vi "test_read-nmea-data2.vi"() -> ()   [LabVIEW 2019] (continued)
F9P\t$GBGSV,1,1,03,11,50,132,,14,87,127,,33,60,219,,3*40\n\t\n15:11:56.71\tF9P\t$GNGLL,3723.52845,N,12656.92271,E,061158.00,A,A*7E\n\t\n15:11:56.73\tF9P\t\t\n15:11:56.75\tF9P\t\t\n15:11:56.77\tF9P\t\t\n15:11:56.79\tF9P\t\t\n15:11:56.81\tF9P\t\t\n15:11:56.83\tF9P\t\t\n15:11:56.85\tF9P\t\t\n15:11:56.87\tF9P\t\t\n15:11:56.89\tF9P\t\t\n15:11:56.91\tF9P\t\t\n15:11:56.93\tF9P\t\t\n15:11:56.95\tF9P\t\t\n15:11:56.97\tF9P\t\t\n15:11:56.99\tF9P\t\t\n15:11:57.01\tF9P\t\t\n15:11:57.03\tF9P\t\t\n15:11:57.05\tF9P\t\t\n15:11:57.07\tF9P\t\t\n15:11:57.09\tF9P\t\t\n15:11:57.11\tF9P\t\t\n15:11:57.13\tF9P\t\t\n15:11:57.15\tF9P\t\t\n15:11:57.17\tF9P\t\t\n15:11:57.19\tF9P\t\t\n15:11:57.21\tF9P\t\t\n15:11:57.23\tF9P\t\t\n15:11:57.25\tF9P\t$GNRMC,061159.00,A,3723.52891,N,12656.92353,E,2.815,44.65,250720,,,A,V*35\n\t\n15:11:57.27\tF9P\t$GNVTG,44.65,T,,M,2.815,N,5.213,K,A*1B\n\t\n15:11:57.29\tF9P\t$GNGGA,061159.00,3723.52891,N,12656.92353,E,1,12,0.67,33.2,M,18.5,M,,*7E\n\t\n15:11:57.31\tF9P\t$GNGSA,A,3,12,06,19,05,17,09,04,02,,,,,1.25,0.67,1.05,1*03\n\t\n15:11:57.33\tF9P\t$GNGSA,A,3,85,70,71,84,,,,,,,,,1.25,0.67,1.05,2*01\n\t\n15:11:57.35\tF9P\t$GNGSA,A,3,36,19,11,04,09,12,,,,,,,1.25,0.67,1.05,3*03\n\t\n15:11:57.37\tF9P\t$GNGSA,A,3,14,11,33,,,,,,,,,,1.25,0.67,1.05,4*02\n\t\n15:11:57.39\tF9P\t$GPGSV,3,1,09,02,55,319,44,04,18,043,20,05,37,247,31,06,64,049,32,1*64\n\t\n15:11:57.41\tF9P\t$GPGSV,3,2,09,09,45,074,39,12,24,277,26,17,33,153,36,19,53,157,32,1*66\n\t\n15:11:57.43\tF9P\t$GPGSV,3,3,09,25,12,307,15,1*59\n\t\n15:11:57.45\tF9P\t$GPGSV,3,1,09,02,55,319,,04,18,043,15,05,37,247,15,06,64,049,26,6*66\n\t\n15:11:57.47\tF9P\t$GPGSV,3,2,09,09,45,074,27,12,24,277,12,17,33,153,25,19,53,157,,6*6A\n\t\n15:11:57.49\tF9P\t$GPGSV,3,3,09,25,12,307,,6*5A\n\t\n15:11:57.51\tF9P\t$GLGSV,2,1,08,69,12,031,,70,71,039,32,71,52,205,43,72,04,209,,1*7C\n\t\n15:11:57.53\tF9P\t$GLGSV,2,2,08,77,01,326,,84,20,122,11,85,70,067,39,86,37,330,,1*72\n\t\n15:11:57.55\tF9P\t$GLGSV,2,1,08,69,12,031,,70,71,039,,71,52,205,28,72,04,209,,3*72\n\t\n15:11:57.57\tF9P\t$GLGSV,2,2,08,77,01,326,,84,20,122,18,85,70,067,24,86,37,330,,3*75\n\t\n15:11:57.59\tF9P\t$GAGSV,2,1,08,02,08,297,10,04,66,118,33,09,32,193,30,11,71,358,24,7*7D\n\t\n15:11:57.61\tF9P\t$GAGSV,2,2,08,12,40,102,31,19,26,045,31,25,09,249,,36,26,308,28,7*73\n\t\n15:11:57.63\tF9P\t$GAGSV,2,1,08,02,08,297,,04,66,118,,09,32,193,26,11,71,358,,2*78\n\t\n15:11:57.65\tF9P\t$GAGSV,2,2,08,12,40,102,,19,26,045,,25,09,249,,36,26,308,,2*7C\n\t\n15:11:57.67\tF9P\t$GBGSV,1,1,03,11,50,132,29,14,87,127,31,33,60,219,38,1*40\n\t\n15:11:57.69\tF9P\t$GBGSV,1,1,03,11,50,132,,14,87,127,31,33,60,219,,3*42\n\t\n15:11:57.71\tF9P\t$GNGLL,3723.52891,N,12656.92353,E,061159.00,A,A*77\n\t\n15:11:57.73\tF9P\t\t\n15:11:57.75\tF9P\t\t\n15:11:57.77\tF9P\t\t\n15:11:57.79\tF9P\t\t\n15:11:57.81\tF9P\t\t\n15:11:57.83\tF9P\t\t\n15:11:57.85\tF9P\t\t\n15:11:57.87\tF9P\t\t\n15:11:57.89\tF9P\t\t\n15:11:57.91\tF9P\t\t\n15:11:57.93\tF9P\t\t\n15:11:57.95\tF9P\t\t\n15:11:57.97\tF9P\t\t\n15:11:57.99\tF9P\t\t\n15:11:58.01\tF9P\t\t\n15:11:58.03\tF9P\t\t\n15:11:58.05\tF9P\t\t\n15:11:58.07\tF9P\t\t\n15:11:58.09\tF9P\t\t\n15:11:58.11\tF9P\t\t\n15:11:58.13\tF9P\t\t\n15:11:58.15\tF9P\t\t\n15:11:58.17\tF9P\t\t\n15:11:58.19\tF9P\t\t\n15:11:58.21\tF9P\t\t\n15:11:58.23\tF9P\t\t\n15:11:58.25\tF9P\t$GNRMC,061200.00,A,3723.52933,N,12656.92401,E,2.063,43.37,250720,,,A,V*3A\n\t\n15:11:58.27\tF9P\t$GNVTG,43.37,T,,M,2.063,N,3.820,K,A*1E\n\t\n15:11:58.29\tF9P\t$GNGGA,061200.00,3723.52933,N,12656.92401,E,1,12,0.68,33.6,M,18.5,M,,*73\n\t\n15:11:58.31\tF9P\t$GNGSA,A,3,12,06,19,05,17,09,04,02,,,,,1.27,0.68,1.07,1*0C\n\t\n15:11:58.33\tF9P\t$GNGSA,A,3,85,70,71,84,,,,,,,,,1.27,0.68,1.07,2*0E\n\t\n15:11:58.35\tF9P\t$GNGSA,A,3,36,19,11,04,09,12,,,,,,,1.27,0.68,1.07,3*0C\n\t\n15:11:58.37\tF9P\t$GNGSA,A,3,14,11,33,,,,,,,,,,1.27,0.68,1.07,4*0D\n\t\n15:11:58.39\tF9P\t$GPGSV,3,1,09,02,55,319,43,04,18,043,20,05,37,247,28,06,64,049,30,1*69\n\t\n15:11:58.41\tF9P\t$GPGSV,3,2,09,09,45,074,37,12,24,277,25,17,33,153,28,19,53,157,31,1*67\n\t\n15:11:58.43\tF9P\t$GPGSV,3,3,09,25,12,307,17,1*5B\n\t\n15:11:58.45\tF9P\t$GPGSV,3,1,09,02,55,319,,04,18,043,14,05,37,247,14,06,64,049,26,6*66\n\t\n15:11:58.47\tF9P\t$GPGSV,3,2,09,09,45,074,27,12,24,277,14,17,33,153,25,19,53,157,,6*6C\n\t\n15:11:58.49\tF9P\t$GPGSV,3,3,09,25,12,307,,6*5A\n\t\n15:11:58.51\tF9P\t$GLGSV,2,1,08,69,12,031,,70,71,039,31,71,52,205,40,72,04,209,,1*7C\n\t\n15:11:58.53\tF9P\t$GLGSV,2,2,08,77,01,326,,84,20,122,10,85,70,067,36,86,37,330,,1*7C\n\t\n15:11:58.55\tF9P\t$GLGSV,2,1,08,69,12,031,,70,71,039,,71,52,205,26,72,04,209,,3*7C\n\t\n15:11:58.57\tF9P\t$GLGSV,2,2,08,77,01,326,,84,20,122,16,85,70,067,23,86,37,330,,3*7C\n\t\n15:11:58.59\tF9P\t$GAGSV,2,1,08,02,08,297,10,04,66,118,33,09,32,193,31,11,71,358,31,7*78\n\t\n15:11:58.61\tF9P\t$GAGSV,2,2,08,12,40,102,31,19,26,045,30,25,09,249,,36,26,308,27,7*7D\n\t\n15:11:58.63\tF9P\t$GAGSV,2,1,08,02,08,297,,04,66,118,,09,32,193,,11,71,358,,2*7C\n\t\n15:11:58.65\tF9P\t$GAGSV,2,2,08,12,40,102,,19,26,045,,25,09,249,,36,26,308,,2*7C\n\t\n15:11:58.67\tF9P\t$GBGSV,1,1,03,11,50,132,28,14,87,127,28,33,60,219,40,1*46\n\t\n15:11:58.69\tF9P\t$GBGSV,1,1,03,11,50,132,,14,87,127,30,33,60,219,,3*43\n\t\n15:11:58.71\tF9P\t$GNGLL,3723.52933,N,12656.92401,E,061200.00,A,A*71\n\t\n15:11:58.73\tF9P\t\t\n15:11:58.75\tF9P\t\t\n15:11:58.77\tF9P\t\t\n15:11:58.79\tF9P\t\t\n15:11:58.81\tF9P\t\t\n15:11:58.83\tF9P\t\t\n15:11:58.85\tF9P\t\t\n15:11:58.87\tF9P\t\t\n15:11:58.89\tF9P\t\t\n15:11:58.91\tF9P\t\t\n15:11:58.93\tF9P\t\t\n15:11:58.95\tF9P\t\t\n15:11:58.97\tF9P\t\t\n15:11:58.99\tF9P\t\t\n15:11:59.01\tF9P\t\t\n15:11:59.03\tF9P\t\t\n15:11:59.05\tF9P\t\t\n15:11:59.07\tF9P\t\t\n15:11:59.09\tF9P\t\t\n15:11:59.11\tF9P\t\t\n15:11:59.13\tF9P\t\t\n15:11:59.15\tF9P\t\t\n15:11:59.17\tF9P\t\t\n15:11:59.19\tF9P\t\t\n15:11:59.21\tF9P\t\t\n15:11:59.23\tF9P\t\t\n15:11:59.25\tF9P\t$GNRMC,061201.00,A,3723.52964,N,12656.92469,E,2.580,59.46,250720,,,A,V*32\n\t\n15:11:59.27\tF9P\t$GNVTG,59.46,T,,M,2.580,N,4.779,K,A*1F\n\t\n15:11:59.29\tF9P\t$GNGGA,061201.00,3723.52964,N,12656.92469,E,1,12,0.73,33.3,M,18.5,M,,*71\n\t\n15:11:59.32\tF9P\t$GNGSA,A,3,12,06,19,05,17,09,02,,,,,,1.41,0.73,1.20,1*07\n\t\n15:11:59.34\tF9P\t$GNGSA,A,3,85,70,71,84,,,,,,,,,1.41,0.73,1.20,2*01\n\t\n15:11:59.36\tF9P\t$GNGSA,A,3,36,19,11,04,09,12,,,,,,,1.41,0.73,1.20,3*03\n\t\n15:11:59.38\tF9P\t$GNGSA,A,3,14,11,33,,,,,,,,,,1.41,0.73,1.20,4*02\n\t\n15:11:59.40\tF9P\t$GPGSV,3,1,09,02,55,319,41,04,18,043,19,05,37,247,27,06,64,049,25,1*6A\n\t\n15:11:59.42\tF9P\t$GPGSV,3,2,09,09,45,074,32,12,24,277,24,17,33,153,36,19,53,157,27,1*6B\n\t\n15:11:59.44\tF9P\t$GPGSV,3,3,09,25,12,307,15,1*59\n\t\n15:11:59.46\tF9P\t$GPGSV,3,1,09,02,55,319,,04,18,043,,05,37,247,,06,64,049,24,6*64\n\t\n15:11:59.48\tF9P\t$GPGSV,3,2,09,09,45,074,27,12,24,277,14,17,33,153,23,19,53,157,,6*6A\n\t\n15:11:59.50\tF9P\t$GPGSV,3,3,09,25,12,307,,6*5A\n\t\n15:11:59.52\tF9P\t$GLGSV,2,1,08,69,12,031,,70,71,039,25,71,52,205,44,72,04,209,,1*7D\n\t\n15:11:59.54\tF9P\t$GLGSV,2,2,08,77,01,326,,84,20,122,14,85,70,067,29,86,37,330,,1*76\n\t\n15:11:59.56\tF9P\t$GLGSV,2,1,08,69,12,031,,70,71,039,,71,52,205,26,72,04,209,,3*7C\n\t\n15:11:59.58\tF9P\t$GLGSV,2,2,08,77,01,326,,84,20,122,11,85,70,067,21,86,37,330,,3*79\n\t\n15:11:59.60\tF9P\t$GAGSV,2,1,08,02,08,297,09,04,66,118,30,09,32,193,35,11,71,358,34,7*72\n\t\n15:11:59.62\tF9P\t$GAGSV,2,2,08,12,40,102,31,19,26,045,29,25,09,249,,36,26,308,26,7*74\n\t\n15:11:59.64\tF9P\t$GAGSV,2,1,08,02,08,297,,04,66,118,,09,32,193,,11,71,358,,2*7C\n\t\n15:11:59.66\tF9P\t$GAGSV,2,2,08,12,40,102,,19,26,045,,25,09,249,,36,26,308,,2*7C\n\t\n15:11:59.68\tF9P\t$GBGSV,1,1,03,11,50,132,20,14,87,127,28,33,60,219,39,1*40\n\t\n15:11:59.70\tF9P\t$GBGSV,1,1,03,11,50,132,,14,87,127,31,33,60,219,,3*42\n\t\n15:11:59.72\tF9P\t$GNGLL,3723.52964,N,12656.92469,E,061201.00,A,A*7C\n\t\n15:11:59.74\tF9P\t\t\n15:11:59.76\tF9P\t\t\n15:11:59.78\tF9P\t\t\n15:11:59.80\tF9P\t\t\n15:11:59.82\tF9P\t\t\n15:11:59.84\tF9P\t\t\n15:11:59.86\tF9P\t\t\n15:11:59.88\tF9P\t\t\n15:11:59.90\tF9P\t\t\n15:11:59.92\tF9P\t\t\n15:11:59.94\tF9P\t\t\n15:11:59.96\tF9P\t\t\n15:11:59.98\tF9P\t\t\n15:12:00.00\tF9P\t\t\n15:12:00.02\tF9P\t\t\n15:12:00.04\tF9P\t\t\n15:12:00.06\tF9P\t\t\n15:12:00.08\tF9P\t\t\n15:12:00.10\tF9P\t\t\n15:12:00.12\tF9P\t\t\n15:12:00.14\tF9P\t\t\n15:12:00.16\tF9P\t\t\n15:12:00.18\tF9P\t\t\n15:12:00.20\tF9P\t\t\n15:12:00.22\tF9P\t\t\n15:12:00.24\tF9P\t\t\n15:12:00.26\tF9P\t$GNRMC,061202.00,A,3723.53000,N,12656.92524,E,2.015,53.71,250720,,,A,V*34\n\t\n15:12:00.28\tF9P\t$GNVTG,53.71,T,,M,2.015,N,3.732,K,A*10\n\t\n15:12:00.30\tF9P\t$GNGGA,061202.00,3723.53000,N,12656.92524,E,1,12,0.70,33.1,M,18.5,M,,*71\n\t\n15:12:00.32\tF9P\t$GNGSA,A,3,12,06,19,05,17,09,04,02,,,,,1.27,0.70,1.06,1*04\n\t\n15:12:00.34\tF9P\t$GNGSA,A,3,85,70,71,84,,,,,,,,,1.27,0.70,1.06,2*06\n\t\n15:12:00.36\tF9P\t$GNGSA,A,3,36,19,11,04,09,12,,,,,,,1.27,0.70,1.06,3*04\n\t\n15:12:00.38\tF9P\t$GNGSA,A,3,14,11,33,,,,,,,,,,1.27,0.70,1.06,4*05\n\t\n15:12:00.40\tF9P\t$GPGSV,3,1,09,02,55,319,43,04,18,043,21,05,37,247,26,06,64,049,31,1*67\n\t\n15:12:00.42\tF9P\t$GPGSV,3,2,09,09,45,074,35,12,24,277,27,17,33,153,37,19,53,157,28,1*61\n\t\n15:12:00.44\tF9P\t$GPGSV,3,3,09,25,12,307,15,1*59\n\t\n15:12:00.46\tF9P\t$GPGSV,3,1,09,02,55,319,,04,18,043,,05,37,247,,06,64,049,23,6*63\n\t\n15:12:00.48\tF9P\t$GPGSV,3,2,09,09,45,074,27,12,24,277,11,17,33,153,23,19,53,157,,6*6F\n\t\n15:12:00.50\tF9P\t$GPGSV,3,3,09,25,12,307,,6*5A\n\t\n15:12:00.52\tF9P\t$GLGSV,2,1,08,69,12,031,,70,71,039,26,71,52,205,42,72,04,209,28,1*72\n\t\n15:12:00.54\tF9P\t$GLGSV,2,2,08,77,01,326,,84,20,122,08,85,70,067,34,86,37,330,,1*77\n\t\n15:12:00.56\tF9P\t$GLGSV,2,1,08,69,12,031,,70,71,039,,71,52,205,25,72,04,209,,3*7F\n\t\n15:12:00.58\tF9P\t$GLGSV,2,2,08,77,01,326,,84,20,122,11,85,70,067,21,86,37,330,,3*79\n\t\n15:12:00.60\tF9P\t$GAGSV,2,1,08,02,08,297,13,04,66,118,33,09,32,193,36,11,71,358,26,7*7A\n\t\n15:12:00.62\tF9P\t$GAGSV,2,2,08,12,40,102,27,19,26,045,28,25,09,249,,36,26,308,25,7*71\n\t\n15:12:00.64\tF9P\t$GAGSV,2,1,08,02,08,297,,04,66,118,,09,32,193,,11,71,358,,2*7C\n\t\n15:12:00.66\tF9P\t$GAGSV,2,2,08,12,40,102,,19,26,045,,25,09,249,,36,26,308,,2*7C\n\t\n15:12:00.68\tF9P\t$GBGSV,1,1,03,11,50,132,31,14,87,127,28,33,60,219,40,1*4E\n\t\n15:12:00.70\tF9P\t$GBGSV,1,1,03,11,50,132,,14,87,127,28,33,60,219,,3*4A\n\t\n15:12:00.72\tF9P\t$GNGLL,3723.53000,N,12656.92524,E,061202.00,A,A*7D\n\t\n15:12:00.74\tF9P\t\t\n15:12:00.76\tF9P\t\t\n15:12:00.78\tF9P\t\t\n15:12:00.80\tF9P\t\t\n15:12:00.82\tF9P\t\t\n15:12:00.84\tF9P\t\t\n15:12:00.86\tF9P\t\t\n15:12:00.88\tF9P\t\t\n15:12:00.90\tF9P\t\t\n15:12:00.92\tF9P\t\t\n15:12:00.94\tF9P\t\t\n15:12:00.96\tF9P\t\t\n15:12:00.98\tF9P\t\t\n15:12:01.00\tF9P\t\t\n15:12:01.02\tF9P\t\t\n15:12:01.04\tF9P\t\t\n15:12:01.06\tF9P\t\t\n15:12:01.08\tF9P\t\t\n15:12:01.10\tF9P\t\t\n15:12:01.12\tF9P\t\t\n15:12:01.14\tF9P\t\t\n15:12:01.16\tF9P\t\t\n15:12:01.18\tF9P\t\t\n15:12:01.20\tF9P\t\t\n15:12:01.22\tF9P\t\t\n15:12:01.24\tF9P\t\t\n15:12:01.26\tF9P\t$GNRMC,061203.00,A,3723.53041,N,12656.92573,E,2.202,48.58,250720,,,A,V*37\n\t\n15:12:01.28\tF9P\t$GNVTG,48.58,T,,M,2.202,N,4.077,K,A*14\n\t\n15:12:01.30\tF9P\t$GNGGA,061203.00,3723.53041,N,12656.92573,E,1,12,0.70,33.4,M,18.5,M,,*72\n\t\n15:12:01.32\tF9P\t$GNGSA,A,3,12,06,19,05,17,09,04,02,,,,,1.27,0.70,1.06,1*04\n\t\n15:12:01.34\tF9P\t$GNGSA,A,3,85,70,71,84,,,,,,,,,1.27,0.70,1.06,2*06\n\t\n15:12:01.36\tF9P\t$GNGSA,A,3,36,19,11,04,09,12,,,,,,,1.27,0.70,1.06,3*04\n\t\n15:12:01.38\tF9P\t$GNGSA,A,3,14,11,33,,,,,,,,,,1.27,0.70,1.06,4*05\n\t\n15:12:01.40\tF9P\t$GPGSV,3,1,09,02,55,319,42,04,18,043,21,05,37,247,30,06,64,049,30,1*60\n\t\n15:12:01.42\tF9P\t$GPGSV,3,2,09,09,45,074,33,12,24,277,27,17,33,153,32,19,53,157,30,1*6B\n\t\n15:12:01.44\tF9P\t$GPGSV,3,3,09,25,12,307,12,1*5E\n\t\n15:12:01.46\tF9P\t$GPGSV,3,1,09,02,55,319,,04,18,043,,05,37,247,,06,64,049,23,6*63\n\t\n15:12:01.48\tF9P\t$GPGSV,3,2,09,09,45,074,32,12,24,277,12,17,33,153,23,19,53,157,,6*68\n\t\n15:12:01.50\tF9P\t$GPGSV,3,3,09,25,12,307,,6*5A\n\t\n15:12:01.52\tF9P\t$GLGSV,2,1,08,69,12,031,,70,71,039,27,71,52,205,44,72,04,209,20,1*7D\n\t\n15:12:01.54\tF9P\t$GLGSV,2,2,08,77,01,326,,84,20,122,11,85,70,067,28,86,37,330,,1*72\n\t\n15:12:01.56\tF9P\t$GLGSV,2,1,08,69,12,031,,70,71,039,,71,52,205,26,72,04,209,,3*7C\n\t\n15:12:01.58\tF9P\t$GLGSV,2,2,08,77,01,326,,84,20,122,08,85,70,067,21,86,37,330,,3*71\n\t\n15:12:01.60\tF9P\t$GAGSV,2,1,08,02,08,297,11,04,66,118,29,09,32,193,37,11,71,358,31,7*74\n\t\n15:12:01.62\tF9P\t$GAGSV,2,2,08,12,40,102,26,19,26,045,28,25,09,249,,36,26,308,23,7*76\n\t\n15:12:01.64\tF9P\t$GAGSV,2,1,08,02,08,297,,04,66,118,,09,32,193,28,11,71,358,,2*76\n\t\n15:12:01.66\tF9P\t$GAGSV,2,2,08,12,40,102,,19,26,045,,25,09,249,,36,26,308,,2*7C\n\t\n15:12:01.68\tF9P\t$GBGSV,1,1,03,11,50,132,25,14,87,127,26,33,60,219,35,1*47\n\t\n15:12:01.70\tF9P\t$GBGSV,1,1,03,11,50,132,,14,87,127,27,33,60,219,,3*45\n\t\n15:12:01.72\tF9P\t$GNGLL,3723.53041,N,12656.92573,E,061203.00,A,A*7B\n\t\n15:12:01.74\tF9P\t\t\n15:12:01.76\tF9P\t\t\n15:12:01.78\tF9P\t\t\n15:12:01.80\tF9P\t\t\n15:12:01.82\tF9P\t\t\n15:12:01.84\tF9P\t\t\n15:12:01.86\tF9P\t\t\n15:12:01.88\tF9P\t\t\n15:12:01.90\tF9P\t\t\n15:12:01.92\tF9P\t\t\n15:12:01.94\tF9P\t\t\n15:12:01.96\tF9P\t\t\n15:12:01.98\tF9P\t\t\n15:12:02.00\tF9P\t\t\n15:12:02.02\tF9P\t\t\n15:12:02.04\tF9P\t\t\n15:12:02.06\tF9P\t\t\n15:12:02.08\tF9P\t\t\n15:12:02.10\tF9P\t\t\n15:12:02.12\tF9P\t\t\n15:12:02.14\tF9P\t\t\n15:12:02.16\tF9P\t\t\n15:12:02.18\tF9P\t\t\n15:12:02.20\tF9P\t\t\n15:12:02.22\tF9P\t\t\n15:12:02.24\tF9P\t\t\n15:12:02.26\tF9P\t$GNRMC,061204.00,A,3723.53076,N,12656.92627,E,2.102,51.21,250720,,,A,V*33\n\t\n15:12:02.28\tF9P\t$GNVTG,51.21,T,,M,2.102,N,3.892,K,A*15\n\t\n15:12:02.30\tF9P\t$GNGGA,061204.00,3723.53076,N,12656.92627,E,1,12,0.76,33.3,M,18.5,M,,*72\n\t\n15:12:02.32\tF9P\t$GNGSA,A,3,12,06,19,05,17,09,04,02,,,,,1.38,0.76,1.15,1*0E\n\t\n15:12:02.34\tF9P\t$GNGSA,A,3,85,70,71,84,,,,,,,,,1.38,0.76,1.15,2*0C\n\t\n15:12:02.36\tF9P\t$GNGSA,A,3,36,19,11,04,09,12,,,,,,,1.38,0.76,1.15,3*0E\n\t\n15:12:02.38\tF9P\t$GNGSA,A,3,14,11,33,,,,,,,,,,1.38,0.76,1.15,4*0F\n\t\n15:12:02.40\tF9P\t$GPGSV,3,1,09,02,55,319,35,04,18,043,20,05,37,247,25,06,64,049,32,1*67\n\t\n15:12:02.42\tF9P\t$GPGSV,3,2,09,09,45,074,33,12,23,276,25,17,33,153,32,19,53,157,34,1*6B\n\t\n15:12:02.44\tF9P\t$GPGSV,3,3,09,25,12,307,13,1*5F\n\t\n15:12:02.46\tF9P\t$GPGSV,3,1,09,02,55,319,,04,18,043,,05,37,247,,06,64,049,23,6*63\n\t\n15:12:02.48\tF9P\t$GPGSV,3,2,09,09,45,074,32,12,23,276,,17,33,153,22,19,53,157,,6*6C\n\t\n15:12:02.50\tF9P\t$GPGSV,3,3,09,25,12,307,,6*5A\n\t\n15:12:02.52\tF9P\t$GLGSV,2,1,08,69,12,031,,70,71,039,27,71,52,205,40,72,04,209,21,1*78\n\t\n15:12:02.54\tF9P\t$GLGSV,2,2,08,77,01,326,,84,20,122,10,85,70,067,32,86,37,330,,1*78\n\t\n15:12:02.56\tF9P\t$GLGSV,2,1,08,69,12,031,,70,71,039,,71,52,205,25,72,04,209,,3*7F\n\t\n15:12:02.58\tF9P\t$GLGSV,2,2,08,77,01,326,,84,20,122,13,85,70,067,21,86,37,330,,3*7B\n\t\n15:12:02.60\tF9P\t$GAGSV,2,1,08,02,08,297,08,04,66,118,28,09,32,193,38,11,71,358,31,7*72\n\t\n15:12:02.62\tF9P\t$GAGSV,2,2,08,12,40,102,27,19,26,045,26,25,09,249,,36,26,308,22,7*78\n\t\n15:12:02.64\tF9P\t$GAGSV,2,1,08,02,08,297,,04,66,118,,09,32,193,,11,71,358,,2*7C\n\t\n15:12:02.66\tF9P\t$GAGSV,2,2,08,12,40,102,,19,26,045,,25,09,249,,36,26,308,,2*7C\n\t\n15:12:02.68\tF9P\t$GBGSV,1,1,03,11,50,132,26,14,87,127,31,33,60,219,33,1*44\n\t\n15:12:02.70\tF9P\t$GBGSV,1,1,03,11,50,132,,14,87,127,,33,60,219,,3*40\n\t\n15:12:02.72\tF9P\t$GNGLL,3723.53076,N,12656.92627,E,061204.00,A,A*7A\n\t\n15:12:02.74\tF9P\t\t\n15:12:02.76\tF9P\t\t\n15:12:02.78\tF9P\t\t\n15:12:02.80\tF9P\t\t\n15:12:02.82\tF9P\t\t\n15:12:02.84\tF9P\t\t\n15:12:02.86\tF9P\t\t\n15:12:02.88\tF9P\t\t\n15:12:02.90\tF9P\t\t\n15:12:02.92\tF9P\t\t\n15:12:02.94\tF9P\t\t\n15:12:02.96\tF9P\t\t\n15:12:02.98\tF9P\t\t\n15:12:03.00\tF9P\t\t\n15:12:03.02\tF9P\t\t\n15:12:03.04\tF9P\t\t\n15:12:03.06\tF9P\t\t\n15:12:03.08\tF9P\t\t\n15:12:03.10\tF9P\t\t\n15:12:03.12\tF9P\t\t\n15:12:03.14\tF9P\t\t\n15:12:03.16\tF9P\t\t\n15:12:03.18\tF9P\t\t\n15:12:03.20\tF9P\t\t\n15:12:03.22\tF9P\t\t\n15:12:03.24\tF9P\t$GNRMC,061205.00,A,3723.53127,N,12656.92691,E,2.614,49.90,250720,,,A,V*39\n\t\n15:12:03.26\tF9P\t$GNVTG,49.90,T,,M,2.614,N,4.840,K,A*1E\n\t\n15:12:03.28\tF9P\t$GNGGA,061205.00,3723.53127,N,12656.92691,E,1,12,0.83,33.5,M,18.5,M,,*77\n\t\n15:12:03.30\tF9P\t$GNGSA,A,3,12,06,19,05,17,09,04,02,,,,,1.56,0.83,1.32,1*09\n\t\n15:12:03.32\tF9P\t$GNGSA,A,3,85,70,71,84,,,,,,,,,1.56,0.83,1.32,2*0B\n\t\n15:12:03.34\tF9P\t$GNGSA,A,3,36,19,11,04,09,12,,,,,,,1.56,0.83,1.32,3*09\n\t\n15:12:03.36\tF9P\t$GNGSA,A,3,14,11,33,,,,,,,,,,1.56,0.83,1.32,4*08\n\t\n15:12:03.38\tF9P\t$GPGSV,3,1,09,02,55,319,40,04,18,043,22,05,37,247,31,06,64,049,34,1*64\n\t\n15:12:03.40\tF9P\t$GPGSV,3,2,09,09,45,074,36,12,23,276,25,17,33,153,36,19,53,157,34,1*6A\n\t\n15:12:03.42\tF9P\t$GPGSV,3,3,09,25,12,307,12,1*5E\n\t\n15:12:03.44\tF9P\t$GPGSV,3,1,09,02,55,319,,04,18,043,,05,37,247,,06,64,049,25,6*65\n\t\n15:12:03.46\tF9P\t$GPGSV,3,2,09,09,45,074,26,12,23,276,,17,33,153,22,19,53,157,,6*69\n\t\n15:12:03.48\tF9P\t$GPGSV,3,3,09,25,12,307,,6*5A\n\t\n15:12:03.50\tF9P\t$GLGSV,2,1,08,69,12,031,,70,71,039,33,71,52,205,39,72,04,209,22,1*70\n\t\n15:12:03.52\tF9P\t$GLGSV,2,2,08,77,01,326,,84,20,122,09,85,70,067,39,86,37,330,,1*7B\n\t\n15:12:03.54\tF9P\t$GLGSV,2,1,08,69,12,031,,70,71,039,,71,52,205,25,72,04,209,,3*7F\n\t\n15:12:03.56\tF9P\t$GLGSV,2,2,08,77,01,326,,84,20,122,07,85,70,067,21,86,37,330,,3*7E\n\t\n15:12:03.58\tF9P\t$GAGSV,2,1,08,02,08,297,10,04,66,118,27,09,32,193,32,11,71,358,31,7*7E\n\t\n15:12:03.60\tF9P\t$GAGSV,2,2,08,12,40,102,31,19,26,045,23,25,09,249,,36,26,308,19,7*72\n\t\n15:12:03.62\tF9P\t$GAGSV,2,1,08,02,08,297,,04,66,118,,09,32,193,33,11,71,358,,2*7C\n\t\n15:12:03.64\tF9P\t$GAGSV,2,2,08,12,40,102,,19,26,045,,25,09,249,,36,26,308,,2*7C\n\t\n15:12:03.66\tF9P\t$GBGSV,1,1,03,11,50,132,31,14,87,127,27,33,60,219,29,1*4E\n\t\n15:12:03.68\tF9P\t$GBGSV,1,1,03,11,50,132,,14,87,127,,33,60,219,,3*40\n\t\n15:12:03.70\tF9P\t$GNGLL,3723.53127,N,12656.92691,E,061205.00,A,A*73\n\t\n15:12:03.72\tF9P\t\t\n15:12:03.74\tF9P\t\t\n15:12:03.76\tF9P\t\t\n15:12:03.78\tF9P\t\t\n15:12:03.80\tF9P\t\t\n15:12:03.82\tF9P\t\t\n15:12:03.84\tF9P\t\t\n15:12:03.86\tF9P\t\t\n15:12:03.88\tF9P\t\t\n15:12:03.90\tF9P\t\t\n15:12:03.92\tF9P\t\t\n15:12:03.94\tF9P\t\t\n15:12:03.96\tF9P\t\t\n15:12:03.98\tF9P\t\t\n15:12:04.00\tF9P\t\t\n15:12:04.02\tF9P\t\t\n15:12:04.04\tF9P\t\t\n15:12:04.06\tF9P\t\t\n15:12:04.08\tF9P\t\t\n15:12:04.10\tF9P\t\t\n15:12:04.12\tF9P\t\t\n15:12:04.14\tF9P\t\t\n15:12:04.16\tF9P\t\t\n15:12:04.18\tF9P\t\t\n15:12:04.20\tF9P\t\t\n15:12:04.22\tF9P\t\t\n15:12:04.24\tF9P\t$GNRMC,061206.00,A,3723.53162,N,12656.92763,E,2.170,51.29,250720,,,A,V*39\n\t\n15:12:04.26\tF9P\t$GNVTG,51.29,T,,M,2.170,N,4.020,K,A*1E\n\t\n15:12:04.28\tF9P\t$GNGGA,061206.00,3723.53162,N,12656.92763,E,1,12,0.87,35.0,M,18.5,M,,*7E\n\t\n15:12:04.30\tF9P\t$GNGSA,A,3,12,06,19,05,17,09,04,02,,,,,1.60,0.87,1.34,1*0E\n\t\n15:12:04.32\tF9P\t$GNGSA,A,3,85,70,71,84,,,,,,,,,1.60,0.87,1.34,2*0C\n\t\n15:12:04.34\tF9P\t$GNGSA,A,3,36,19,11,04,09,12,,,,,,,1.60,0.87,1.34,3*0E\n\t\n15:12:04.36\tF9P\t$GNGSA,A,3,14,11,33,,,,,,,,,,1.60,0.87,1.34,4*0F\n\t\n15:12:04.38\tF9P\t$GPGSV,3,1,09,02,55,319,41,04,18,043,26,05,37,247,32,06,64,049,38,1*6E\n\t\n15:12:04.40\tF9P\t$GPGSV,3,2,09,09,45,074,34,12,23,276,22,17,33,153,34,19,53,157,32,1*6B\n\t\n15:12:04.42\tF9P\t$GPGSV,3,3,09,25,12,307,11,1*5D\n\t\n15:12:04.44\tF9P\t$GPGSV,3,1,09,02,55,319,,04,18,043,,05,37,247,26,06,64,049,26,6*62\n\t\n15:12:04.46\tF9P\t$GPGSV,3,2,09,09,45,074,27,12,23,276,22,17,33,153,22,19,53,157,,6*68\n\t\n15:12:04.48\tF9P\t$GPGSV,3,3,09,25,12,307,,6*5A\n\t\n15:12:04.50\tF9P\t$GLGSV,2,1,08,69,12,031,,70,71,039,33,71,52,205,40,72,04,209,22,1*7E\n\t\n15:12:04.52\tF9P\t$GLGSV,2,2,08,77,01,326,,84,20,122,11,85,70,067,42,86,37,330,,1*7E\n\t\n15:12:04.54\tF9P\t$GLGSV,2,1,08,69,12,031,,70,71,039,,71,52,205,24,72,04,209,,3*7E\n\t\n15:12:04.56\tF9P\t$GLGSV,2,2,08,77,01,326,,84,20,122,15,85,70,067,28,86,37,330,,3*74\n
